vi "FTT jpg Display.vi"(8 "error in (no error)":errorcluster caption="错误输入（无错误）", 9 "Model":string, 10 "Roof Picture":refnum<vi>, 11 "Vehicle Picture":refnum<vi>) -> (0 "错误输出":errorcluster)   [LabVIEW 2014]
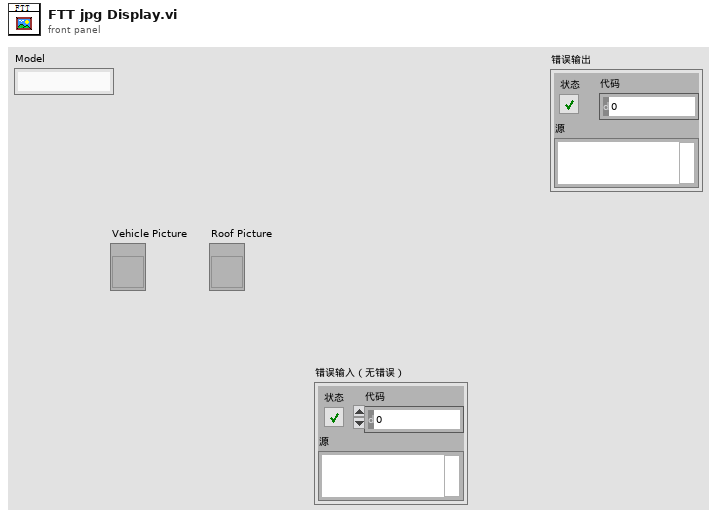
[diagram p1: front panel]
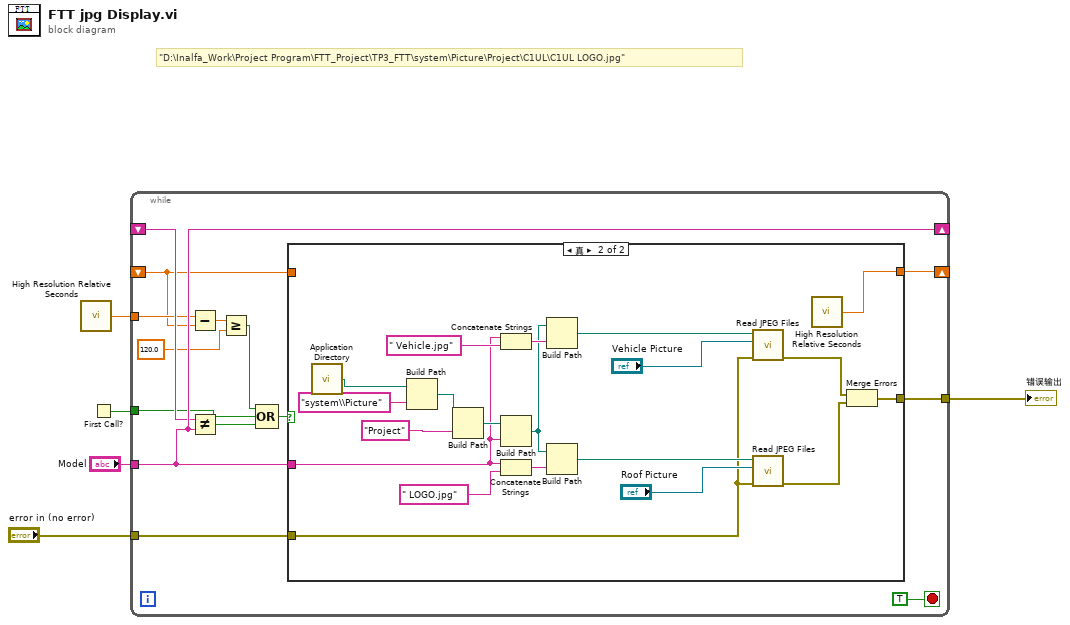
[diagram p0: block diagram]
diagram:
  # "\"D:\\Inalfa_Work\\Project Program\\FTT_Project\\TP3_FTT\\system\\Picture\\Project\\C1UL\\C1UL LOGO.jpg\""
  n1 = call <vilib>:"High Resolution Relative Seconds.vi"() -> ("relative seconds"=w1:dbl)
  n2 = First Call?() -> (First Call?: T/F=w2:bool)
  n3 = while {
    tunnel: [w19] -> w5
    tunnel: "Model" -> [w17]
    shift-right: [w17] -> _
    shift-left: _ -> [w16]
    tunnel: "error in (no error)" -> [w15]
    tunnel: w2 -> [w12]
    shift-right: [w11] -> _
    shift-left: _ -> [w9]
    tunnel: w1 -> [w10]
    stop <- TRUE stop-if-true
    n4 = Subtract(x=w10, y=w9) -> (x-y=w8:dbl)
    n5 = Not Equal?(x=w16, y=w17) -> (x != y?=w14:bool)
    n6 = Greater Or Equal?(x=w8, y=120.0) -> (x >= y?=w7:bool)
    n7 = Compound Arithmetic op=OR(w7, w12, w14) -> (w13:bool)
    n8 = case shown="真" w13 {
      tunnel: [w21 w25] -> w19
      tunnel: w17 -> [_ w24]
      tunnel: w15 -> [w21 w23]
      tunnel: [w20 w22] -> w11
      tunnel: w9 -> [w20 _]
      frame False {
      }
      frame True {
        n9 = call <vilib>:"Application Directory.vi"() -> ("Application Directory"=w41:path)
        n10 = Build Path(base path=w41, name or relative path="system\\Picture") -> (appended path=w39:path)
        n11 = Build Path(base path=w39, name or relative path="Project") -> (appended path=w37:path)
        n12 = Concatenate Strings(w24, " Vehicle.jpg" ("string")) -> (w34:string)
        n13 = Build Path(base path=w37, name or relative path=w24) -> (appended path=w30:path)
        n14 = Concatenate Strings(w24, " LOGO.jpg" ("string")) -> (w33:string)
        n15 = Build Path(base path=w30, name or relative path=w34) -> (appended path=w32:path)
        n16 = Build Path(base path=w30, name or relative path=w33) -> (appended path=w31:path)
        n17 = call "Read JPEG Files.vi"("error in"=w23, "Picture Subpanel"="Vehicle Picture", "JPEG file path"=w32) -> ("error out"=w27:errorcluster)  [unwired: 8 in]
        n18 = call "Read JPEG Files.vi"("error in"=w23, "Picture Subpanel"="Roof Picture", "JPEG file path"=w31) -> ("error out"=w26:errorcluster)  [unwired: 8 in]
        n19 = call <vilib>:"High Resolution Relative Seconds.vi"() -> ("relative seconds"=w22:dbl)
        n20 = Merge Errors(w27, w26) -> (w25:errorcluster)
      }
    }
  }
  "错误输出" <- w5
